vi "get_config_cluster.vi"(8 "error in (no error)":errorcluster, 11 "GenericComponent in":refnum<class "TrajectoryDL090201FrameScan.lvclass">) -> (0 "error out":errorcluster, 2 "config cluster (variant)":variant, 3 "GenericComponent out":refnum<class "TrajectoryDL090201FrameScan.lvclass">)   [LabVIEW 2010, in "TrajectoryDL090201FrameScan.lvclass"]
uses:
  TrajectoryDL090201FrameScan.lvclass
  TrajectoryDL090201FrameScan.lvclass/TrajectoryDL090201FrameScan.ctl
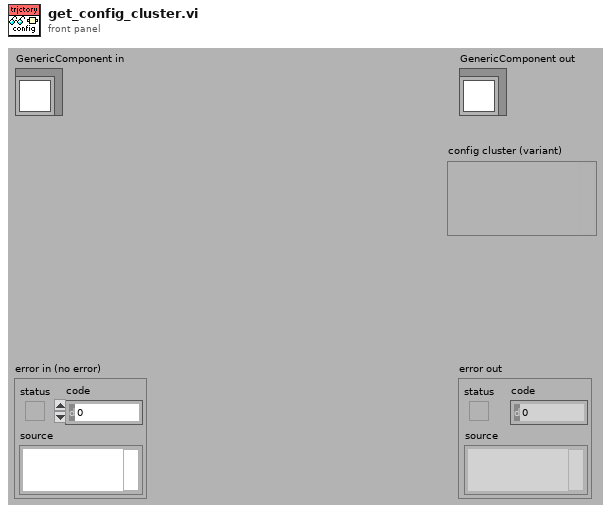
[diagram p1: front panel]
types:
  T1 = typedef "TrajectoryDL090201FrameScan.lvclass/config_cluster.ctl" = cluster{"x scan cut-off fraction":dbl, "x retrace fraction":dbl, "y retrace fraction":dbl}
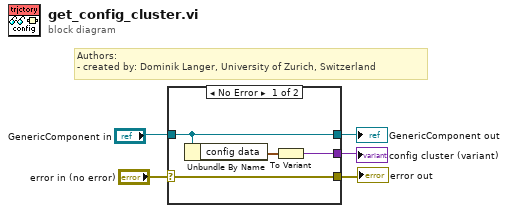
[diagram p0: block diagram]
diagram:
  # "Authors: \n- created by: Dominik Langer, University of Zurich, Switzerland"
  n1 = case shown="No Error" "error in (no error)" {
    selector: "error in (no error)" -> [w9 w10]
    tunnel: "GenericComponent in" -> [w8 w11]
    tunnel: [w9 w10] -> w5
    tunnel: [w8 w11] -> w3
    tunnel: [w6 _] -> w4
    frame No Error {
      n2 = Unbundle By Name(w8) -> ("config data"=w7:T1)
      n3 = To Variant(anything=w7) -> (Variant=w6:variant)
    }
    frame Error {
    }
  }
  "error out" <- w5
  "GenericComponent out" <- w3
  "config cluster (variant)" <- w4
